vi "n load correction file.vi"(0 "n":u16, 1 "ky":dbl, 2 "xoffset":dbl, 5 "filename":string, 7 "cortable":i16, 9 "kx":dbl, 11 "error in (no error)":errorcluster, 12 "phi":dbl, 13 "yoffset":dbl) -> (4 "function return":i16, 15 "error out":errorcluster)   [LabVIEW 2015, in "SCANalone4x64.lvlib"]
doc: "__declspec(dllimport) short __stdcall n_load_correction_file(unsigned short n, const char* filename, short cortable, double kx, double ky, double phi, double xoffset, double yoffset);"
uses:
  <userlib>/SCANalone4x64/SCANalone4x64.lvlib
  <userlib>/SCANalone4x64/SCANalone4x64.dll
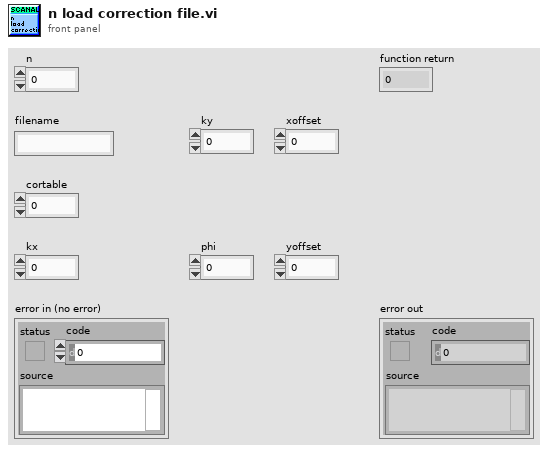
[diagram p1: front panel]
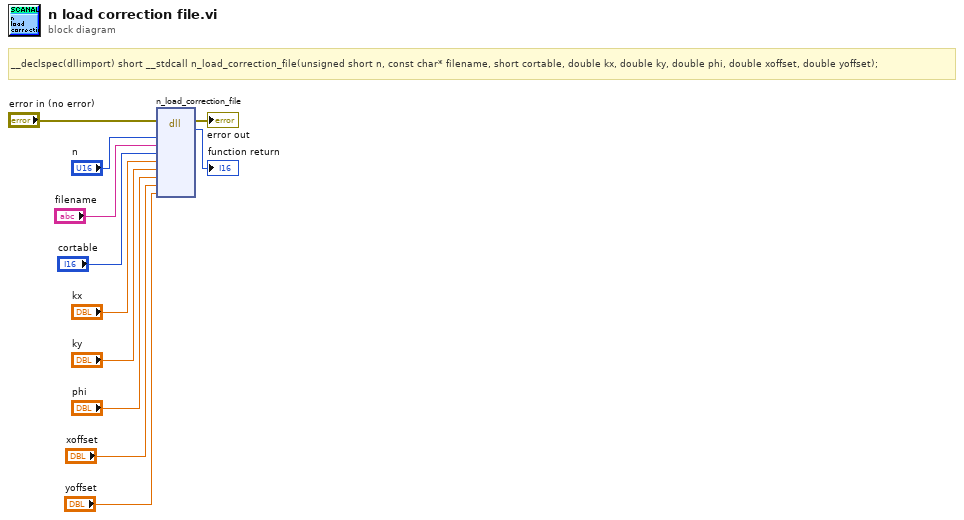
[diagram p0: block diagram]
diagram:
  # "__declspec(dllimport) short __stdcall n_load_correction_file(unsigned short n, const char* filename, short cortable, double kx, double ky, double phi, double xoffset, double yoffset);"
  n1 = dll-call lib="C:/Program Files/National Instruments/LabVIEW 2015/user.lib/SCANalone4x64/SCANalone4x64.*" fn="n_load_correction_file"(error in="error in (no error)", "n"="n", "filename"="filename", "cortable"="cortable", "kx"="kx", "ky"="ky", "phi"="phi", "xoffset"="xoffset", "yoffset"="yoffset") -> (error out=→"error out":errorcluster, →"function return":i16)  [unwired: 10 in, 1 out]
